vi "crosstalkTest.vi"(8 "error in (no error)":errorcluster caption="错误输入（无错误）", 9 "NEXT By Trace":bool, 10 "Channel":string="1", 11 "N5230 输入":refnum<class "N5230.lvclass"> caption="DNL_LabVIEW Object in") -> (0 "error out":errorcluster caption="错误输出", 1 "Data out":dbl[](array[numeric]), 2 "Fre":dbl[](array[numeric]), 3 "N5230 输出":refnum<class "N5230.lvclass"> caption="DNL_LabVIEW Object out")   [LabVIEW 2011, in "N5230.lvclass"]
uses:
  N5230.lvclass
panel:
  in  "VNA Model:":enum16{"E5071C", "N5230A(C)", "N5224A"}(ring)=enum."N5224A"
  in  "VNA VISA":refnum<visa-resource-name>="TCPIP0::A-N5224A-41544.local::hislip0::INSTR"
  out "波形图":dbl[](graph)
  out "Points":i32
  in  "Sample PN:":string="1111111"
  in  "SampleSN:":string="1111111"
  out "dup path":path
  out "Find?":bool
  in  "NEXT By Trace 2":bool
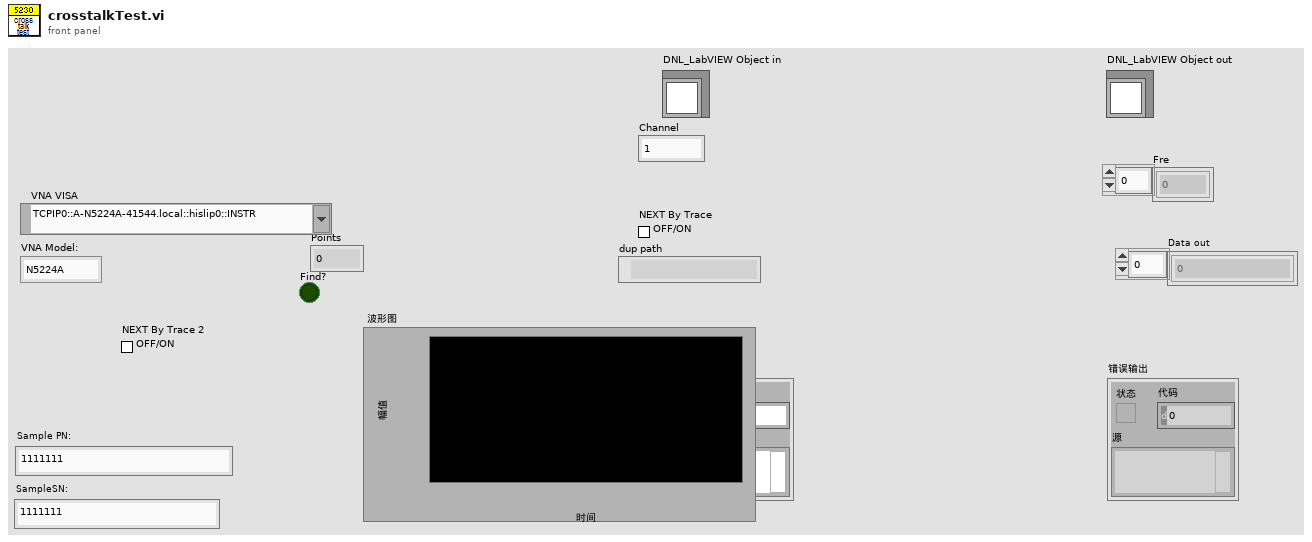
[diagram p1: front panel]
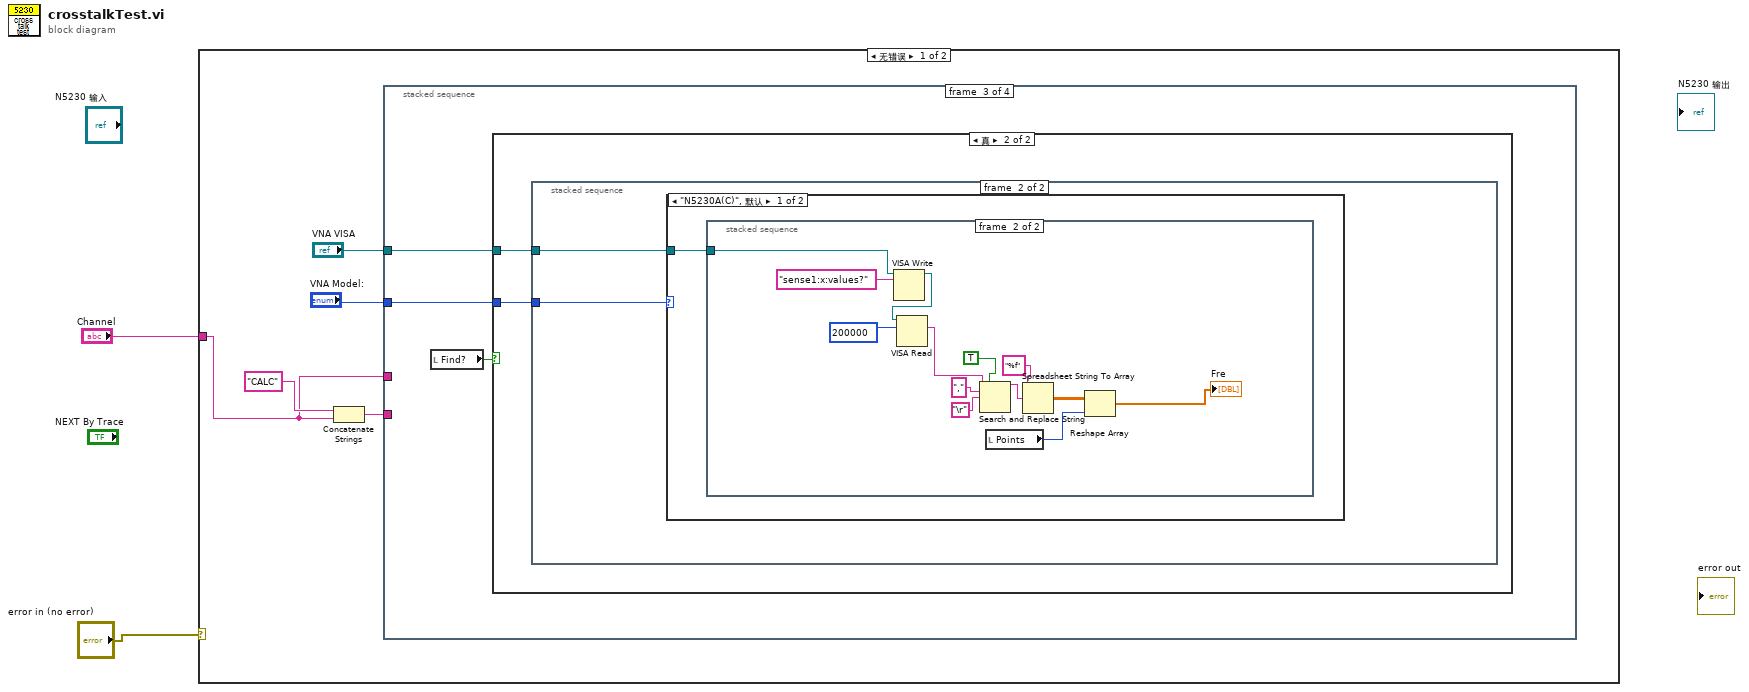
[diagram p0: block diagram]
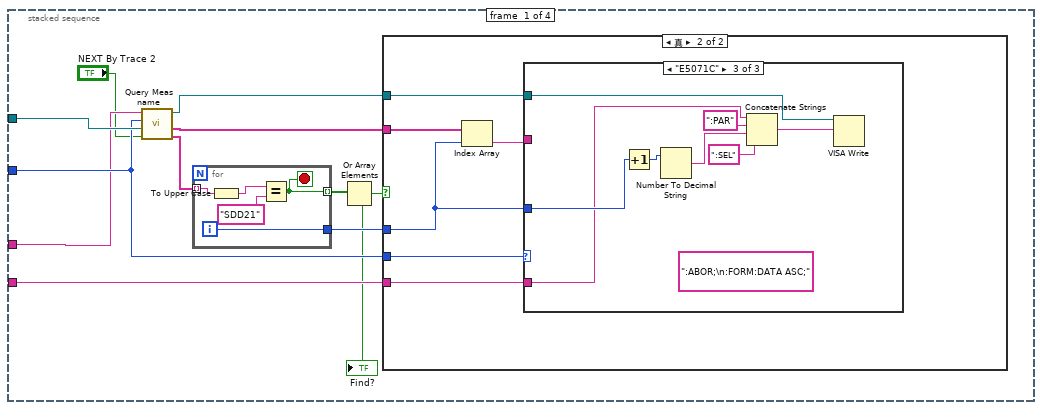
[diagram p2: hidden frame]
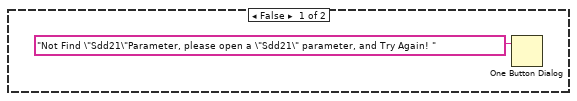
[diagram p3: hidden frame]
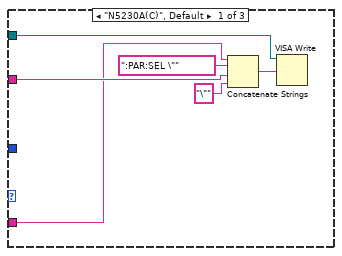
[diagram p4: hidden frame]
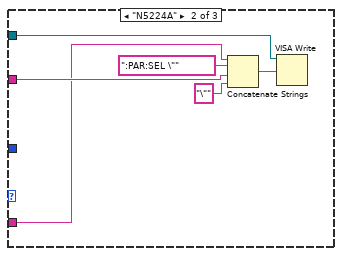
[diagram p5: hidden frame]
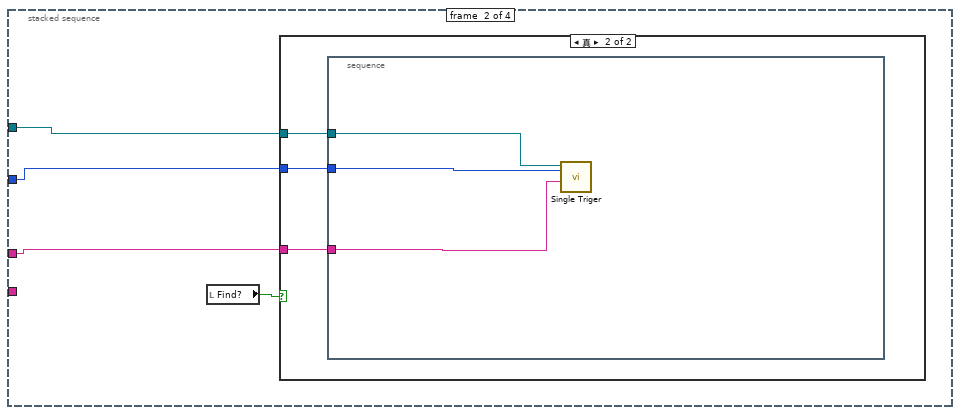
[diagram p6: hidden frame]
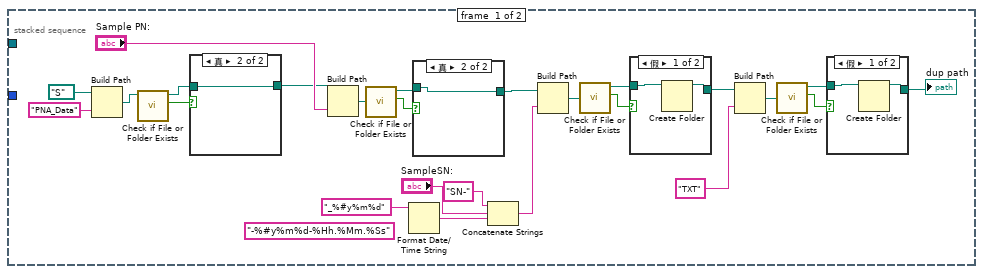
[diagram p9: hidden frame]
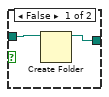
[diagram p12: hidden frame]
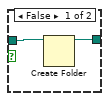
[diagram p13: hidden frame]
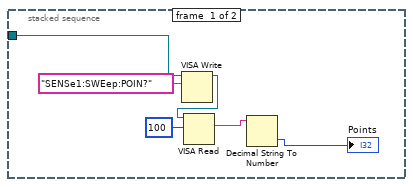
[diagram p14: hidden frame]
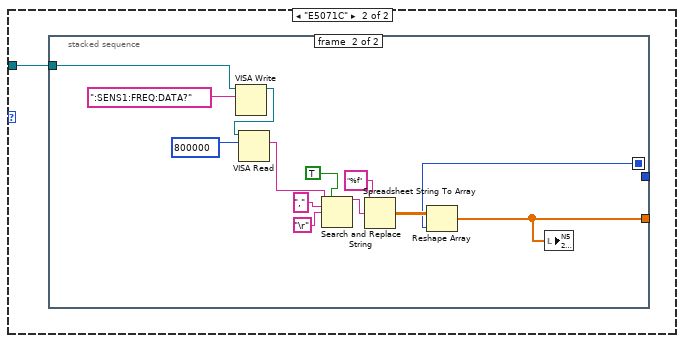
[diagram p15: hidden frame]
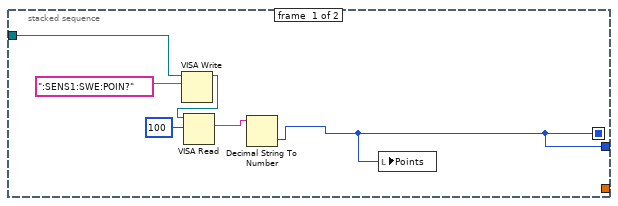
[diagram p16: hidden frame]
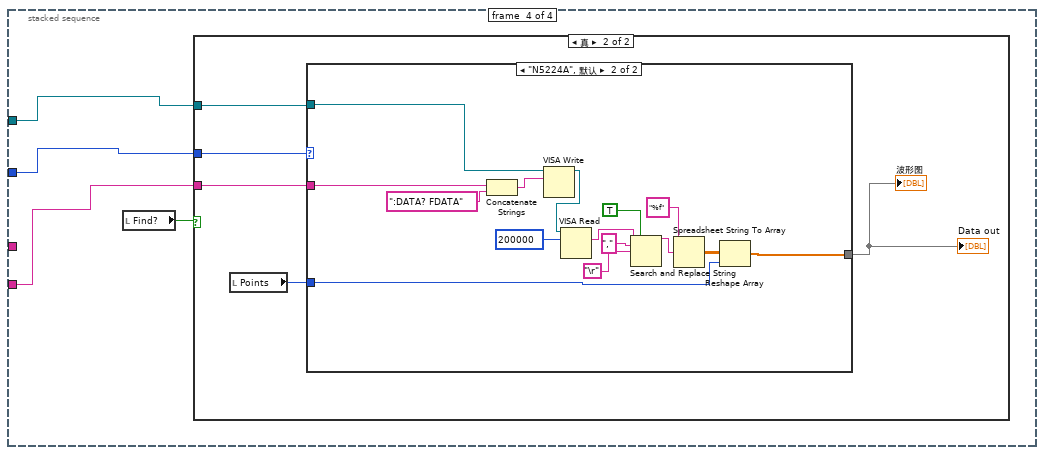
[diagram p17: hidden frame]
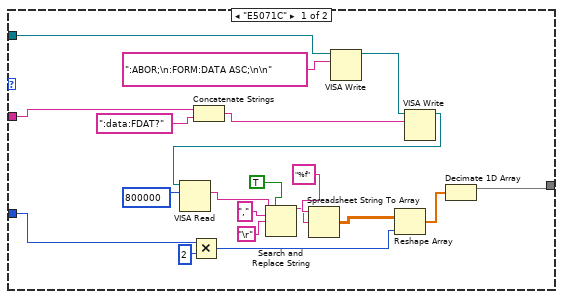
[diagram p19: hidden frame]
diagram:
  n1 = case shown="无错误" "error in (no error)" {
    tunnel: "Channel" -> [w3 _]
    frame No Error {
      n2 = Concatenate Strings("CALC" ("字符串"), w3) -> (w4:string)
      n3 = stacked-sequence {
        tunnel: "VNA VISA" -> [w18 w54 w63 w148]
        tunnel: "VNA Model:" -> [w17 w53 w62 w147]
        tunnel: w4 -> [w15 _ _ w146]
        tunnel: w3 -> [w16 w52 _ _]
        frame #0 {
          n4 = call "Query Meas name.vi"("NEXT By Trace"="NEXT By Trace 2", "VISA resource name"=w18, "VNA Model"=w17, "Channel"=w16) -> ("Parameter item"=w12:string[], "Name list"=w14:string[], "Dup VISA resource name"=w13:refnum<visa-resource-name>)  [unwired: 3 in]
          n5 = for {
            tunnel: w12 -> [w47] mode=indexing
            tunnel: [w50] -> w10 mode=indexing
            tunnel: [w49] -> w11
            i -> [w49]
            stop <- w50 stop-if-true
            n6 = To Upper Case(1:w47) -> (0:w46:string)
            n7 = Equal?(x=w46, y="SDD21") -> (x = y?=w50:bool)
          }
          n8 = Or Array Elements(Boolean array=w10) -> (logical OR=w9:bool)
          "Find?" <- w9
          n9 = case shown="真" w9 {
            tunnel: w14 -> [_ w25]
            tunnel: w13 -> [_ w24]
            tunnel: w17 -> [_ w23]
            tunnel: w15 -> [_ w21]
            tunnel: w11 -> [_ w20]
            frame False {
              n10 = One Button Dialog(message="Not Find \"Sdd21\"Parameter, please open a \"Sdd21\" parameter, and Try Again! " ("消息")) -> ()  [unwired: 1 in, 1 out]
            }
            frame True {
              n11 = Index Array(array=w25, index=w20) -> (element=w22:string)
              n12 = case shown="\"E5071C\"" w23 {
                tunnel: w24 -> [w28 w34 w42]
                tunnel: w22 -> [w27 w33 _]
                tunnel: w20 -> [_ _ w40]
                tunnel: w21 -> [w26 w32 w38]
                frame "N5230A(C)", Default {
                  n13 = Concatenate Strings(w26, ":PAR:SEL \"", w27, "\"" ("string")) -> (w29:string)
                  n14 = VISA Write(VISA resource name=w28, write buffer=w29) -> ()  [unwired: 1 in, 3 out]
                }
                frame "N5224A" {
                  n15 = Concatenate Strings(w32, ":PAR:SEL \"", w33, "\"" ("string")) -> (w35:string)
                  n16 = VISA Write(VISA resource name=w34, write buffer=w35) -> ()  [unwired: 1 in, 3 out]
                }
                frame "E5071C" {
                  (unwired) ":ABOR;\n:FORM:DATA ASC;"
                  n17 = Increment(x=w40) -> (x+1=w41:i32)
                  n18 = Number To Decimal String(number=w41) -> (decimal integer string=w39:string)  [unwired: 1 in]
                  n19 = Concatenate Strings(w38, ":PAR" ("string"), w39, ":SEL" ("string")) -> (w45:string)
                  n20 = VISA Write(VISA resource name=w42, write buffer=w45) -> ()  [unwired: 1 in, 3 out]
                }
              }
            }
          }
        }
        frame #1 {
          n21 = local read "Find?"() -> (w51:bool)
          n22 = case shown="真" w51 {
            tunnel: w54 -> [_ w57]
            tunnel: w53 -> [_ w56]
            tunnel: w52 -> [_ w55]
            frame False {
            }
            frame True {
              n23 = stacked-sequence {
                tunnel: w57 -> [w59]
                tunnel: w56 -> [w60]
                tunnel: w55 -> [w58]
                frame #0 {
                  n24 = call "Single Triger.vi"("Channel"=w58, "VNA Model:"=w60, "VISA"=w59) -> ()  [unwired: 9 in]
                }
              }
            }
          }
        }
        frame #2 {
          n25 = local read "Find?"() -> (w61:bool)
          n26 = case shown="真" w61 {
            tunnel: w63 -> [_ w65]
            tunnel: w62 -> [_ w64]
            frame False {
            }
            frame True {
              n27 = stacked-sequence {
                tunnel: w64 -> [_ w104]
                tunnel: w65 -> [_ w103]
                frame #0 {
                  (unwired) "-%#y%m%d-%Hh.%Mm.%Ss" ("time format string (%c)")
                  n28 = Build Path(base path=path "S:/" ("基路径"), name or relative path="PNA_Data" ("名称或相对路径")) -> (appended path=w74:path)
                  n29 = call <vilib>:"Check if File or Folder Exists.vi"("path"=w74) -> ("file or folder exists?"=w75:bool, "dup path"=w76:path)  [unwired: 8 in, 1 out]
                  n30 = case shown="真" w75 {
                    tunnel: w76 -> [w101 w102]
                    tunnel: [w100 w102] -> w77
                    frame False {
                      n31 = Create Folder(path (use dialog)=w101) -> (created path=w100:path)  [unwired: 2 in, 2 out]
                    }
                    frame True {
                    }
                  }
                  n32 = Build Path(base path=w77, name or relative path="Sample PN:") -> (appended path=w79:path)
                  n33 = call <vilib>:"Check if File or Folder Exists.vi"("path"=w79) -> ("file or folder exists?"=w80:bool, "dup path"=w81:path)  [unwired: 8 in, 1 out]
                  n34 = Format Date/Time String(time format string (%c)="_%#y%m%d") -> (date/time string=w87:string)  [unwired: 2 in]
                  n35 = case shown="真" w80 {
                    tunnel: w81 -> [w98 w99]
                    tunnel: [w97 w99] -> w82
                    frame False {
                      n36 = Create Folder(path (use dialog)=w98) -> (created path=w97:path)  [unwired: 2 in, 2 out]
                    }
                    frame True {
                    }
                  }
                  n37 = Concatenate Strings("SN-" ("字符串"), "SampleSN:", w87) -> (w88:string)
                  n38 = Build Path(base path=w82, name or relative path=w88) -> (appended path=w83:path)
                  n39 = call <vilib>:"Check if File or Folder Exists.vi"("path"=w83) -> ("file or folder exists?"=w85:bool, "dup path"=w84:path)  [unwired: 8 in, 1 out]
                  n40 = case shown="假" w85 {
                    tunnel: w84 -> [w95 w96]
                    tunnel: [w94 w96] -> w67
                    frame False {
                      n41 = Create Folder(path (use dialog)=w95) -> (created path=w94:path)  [unwired: 2 in, 2 out]
                    }
                    frame True {
                    }
                  }
                  n42 = Build Path(base path=w67, name or relative path="TXT" ("名称或相对路径")) -> (appended path=w71:path)
                  n43 = call <vilib>:"Check if File or Folder Exists.vi"("path"=w71) -> ("file or folder exists?"=w69:bool, "dup path"=w70:path)  [unwired: 8 in, 1 out]
                  n44 = case shown="假" w69 {
                    tunnel: w70 -> [w92 w93]
                    tunnel: [w91 w93] -> w68
                    frame False {
                      n45 = Create Folder(path (use dialog)=w92) -> (created path=w91:path)  [unwired: 2 in, 2 out]
                    }
                    frame True {
                    }
                  }
                  "dup path" <- w68
                }
                frame #1 {
                  n46 = case shown="\"N5230A(C)\", 默认" w104 {
                    tunnel: w103 -> [w105 w125]
                    frame "N5230A(C)", Default {
                      n47 = stacked-sequence {
                        tunnel: w105 -> [w108 w114]
                        frame #0 {
                          n48 = VISA Write(VISA resource name=w108, write buffer="SENSe1:SWEep:POIN?") -> (VISA resource name out=w109:refnum<visa-resource-name>)  [unwired: 1 in, 2 out]
                          n49 = VISA Read(VISA resource name=w109, byte count=u32 100) -> (read buffer=w107:string)  [unwired: 1 in, 3 out]
                          n50 = Decimal String To Number(string=w107) -> (number=→"Points":i32)  [unwired: 2 in, 1 out]
                        }
                        frame #1 {
                          n51 = VISA Write(VISA resource name=w114, write buffer="sense1:x:values?") -> (VISA resource name out=w123:refnum<visa-resource-name>)  [unwired: 1 in, 2 out]
                          n52 = VISA Read(VISA resource name=w123, byte count=u32 200000) -> (read buffer=w122:string)  [unwired: 1 in, 3 out]
                          n53 = Search and Replace String(replace all?=TRUE ("replace all? (F)"), input string=w122, search string=",", replace string="\r") -> (result string=w118:string)  [unwired: 4 in, 3 out]
                          n54 = local read "Points"() -> (w113:i32)
                          n55 = Spreadsheet String To Array(format string="%f", spreadsheet string=w118) -> (array=w121:dbl[][])  [unwired: 2 in]
                          n56 = Reshape Array(w121, w113) -> (→"Fre":dbl[])
                        }
                      }
                    }
                    frame "E5071C" {
                      n57 = stacked-sequence {
                        seq-local: [w126 _] -> [_ w134]
                        tunnel: w125 -> [w129 w135]
                        tunnel: [_ w132] -> _
                        tunnel: [w126 _] -> _
                        frame #0 {
                          n58 = VISA Write(VISA resource name=w129, write buffer=":SENS1:SWE:POIN?") -> (VISA resource name out=w130:refnum<visa-resource-name>)  [unwired: 1 in, 2 out]
                          n59 = VISA Read(VISA resource name=w130, byte count=u32 100) -> (read buffer=w128:string)  [unwired: 1 in, 3 out]
                          n60 = Decimal String To Number(string=w128) -> (number=w126:i32)  [unwired: 2 in, 1 out]
                          n61 = local write "Points"(w126) -> ()
                        }
                        frame #1 {
                          n62 = VISA Write(VISA resource name=w135, write buffer=":SENS1:FREQ:DATA?") -> (VISA resource name out=w144:refnum<visa-resource-name>)  [unwired: 1 in, 2 out]
                          n63 = VISA Read(VISA resource name=w144, byte count=u32 800000) -> (read buffer=w143:string)  [unwired: 1 in, 3 out]
                          n64 = Search and Replace String(replace all?=TRUE ("replace all? (F)"), input string=w143, search string=",", replace string="\r") -> (result string=w139:string)  [unwired: 4 in, 3 out]
                          n65 = Spreadsheet String To Array(format string="%f", spreadsheet string=w139) -> (array=w142:dbl[][])  [unwired: 2 in]
                          n66 = Reshape Array(w142, w134) -> (w132:dbl[])
                          n67 = local write item#-1(w132) -> ()
                        }
                      }
                    }
                  }
                }
              }
            }
          }
        }
        frame #3 {
          n68 = local read "Find?"() -> (w145:bool)
          n69 = case shown="真" w145 {
            tunnel: w147 -> [_ w153]
            tunnel: w148 -> [_ w152]
            tunnel: w146 -> [_ w151]
            frame False {
            }
            frame True {
              n70 = local read "Points"() -> (w150:i32)
              n71 = case shown="\"N5224A\", 默认" w153 {
                tunnel: w152 -> [w157 w175]
                tunnel: [w173 w181] -> w149
                tunnel: w150 -> [w170 w180]
                tunnel: w151 -> [w156 w176]
                frame "E5071C" {
                  n72 = Multiply(x=w170, y=2) -> (x*y=w159:i32)
                  n73 = Concatenate Strings(w156, ":data:FDAT?" ("write buffer")) -> (w154:string)
                  n74 = VISA Write(VISA resource name=w157, write buffer=":ABOR;\n:FORM:DATA ASC;\n\n") -> (VISA resource name out=w171:refnum<visa-resource-name>)  [unwired: 1 in, 2 out]
                  n75 = VISA Write(VISA resource name=w171, write buffer=w154) -> (VISA resource name out=w161:refnum<visa-resource-name>)  [unwired: 1 in, 2 out]
                  n76 = VISA Read(VISA resource name=w161, byte count=u32 800000) -> (read buffer=w168:string)  [unwired: 1 in, 3 out]
                  n77 = Search and Replace String(replace all?=TRUE ("replace all? (F)"), input string=w168, search string=",", replace string="\r") -> (result string=w165:string)  [unwired: 4 in, 3 out]
                  n78 = Spreadsheet String To Array(format string="%f", spreadsheet string=w165) -> (array=w160:dbl[][])  [unwired: 2 in]
                  n79 = Reshape Array(w160, w159) -> (w158:dbl[])
                  n80 = Decimate 1D Array(w158) -> (w173:dbl[])  [unwired: 1 out]
                }
                frame "N5224A", Default {
                  n81 = Concatenate Strings(w176, ":DATA? FDATA" ("write buffer")) -> (w178:string)
                  n82 = VISA Write(VISA resource name=w175, write buffer=w178) -> (VISA resource name out=w183:refnum<visa-resource-name>)  [unwired: 1 in, 2 out]
                  n83 = VISA Read(VISA resource name=w183, byte count=u32 200000) -> (read buffer=w184:string)  [unwired: 1 in, 3 out]
                  n84 = Search and Replace String(replace all?=TRUE ("replace all? (F)"), input string=w184, search string=",", replace string="\r") -> (result string=w187:string)  [unwired: 4 in, 3 out]
                  n85 = Spreadsheet String To Array(format string="%f", spreadsheet string=w187) -> (array=w182:dbl[][])  [unwired: 2 in]
                  n86 = Reshape Array(w182, w180) -> (w181:dbl[])
                }
              }
              "波形图" <- w149
              "Data out" <- w149
            }
          }
        }
      }
    }
    frame Error {
    }
  }
